vi "get data types of channels.vi"(8 "error in (no error)":errorcluster, 11 "channels in":refnum<class "TBM channel.lvclass">[](array[class])) -> (0 "error out":errorcluster, 2 "data types":T1[](array[typedef]), 3 "channels out":refnum<class "TBM channel.lvclass">[](array[class]))   [LabVIEW 2013, in "Shared Memory configuration.lvclass"]
uses:
  Shared Memory configuration.lvclass
  <vilib>/NI/Tag Bus Module Framework/channel/TBM channel.lvclass
  <vilib>/NI/Tag Bus/tag/Data Type.ctl
  <vilib>/NI/Tag Bus/tag/tag descriptor.lvclass/tag descriptor.ctl
  <vilib>/NI/Tag Bus/tag/tag descriptor.lvclass
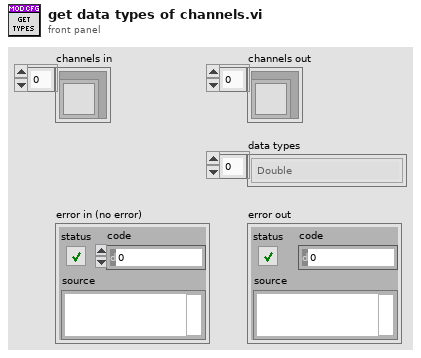
[diagram p1: front panel]
types:
  T1 = typedef "tag bus.lvlib/tag descriptor.lvclass/Data Type.ctl" = enum16{"Double", "Single", "I64", "I32", "I16", "I8", "U64", "U32", "U16", "U8", "Boolean", "String", "Array of Double", "Array of Single", "Array of I64", "Array of I32", "Array of I16", "Array of I8", "Array of U64", "Array of U32", "Array of U16", "Array of U8", "Array of Boolean", "Array of String"}
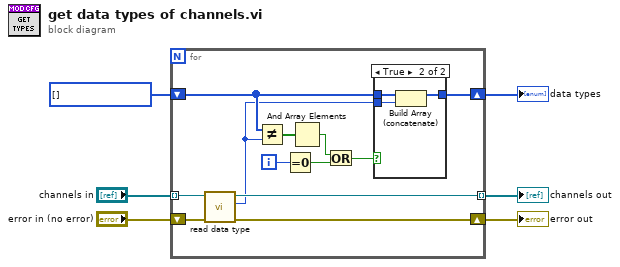
[diagram p0: block diagram]
diagram:
  w2 = T1[] [] items=["Double", "Single", "I64", "I32", "I16", "I8", "U64", "U32", "U16", "U8", "Boolean", "String", "Array of Double", "Array of Single", "Array of I64", "Array of I32", "Array of I16", "Array of I8", "Array of U64", "Array of U32", "Array of U16", "Array of U8", "Array of Boolean", "Array of String"]
  n1 = for {
    tunnel: "channels in" -> [w18] mode=indexing
    shift-right: [w16] -> w4
    shift-left: w2 -> [w15]
    shift-right: [w10] -> w6
    shift-left: "error in (no error)" -> [w9]
    tunnel: [w8] -> w5 mode=indexing
    i -> [w17]
    n2 = call <vilib>:"read data type.vi"("error in"=w9, "system tag in"=w18) -> ("error out"=w10:errorcluster, "data type"=w7:T1, "system tag out"=w8:refnum<class "TBM channel.lvclass">)  [unwired: 7 in]
    n3 = Not Equal?(x=w15, y=w7) -> (x != y?=w14:bool[])
    n4 = Equal To 0?(x=w17) -> (x = 0?=w12:bool)
    n5 = And Array Elements(Boolean array=w14) -> (logical AND=w13:bool)
    n6 = Or(x=w13, y=w12) -> (x .or. y?=w11:bool)
    n7 = case shown="True" w11 {
      tunnel: w15 -> [w19 w22]
      tunnel: [w19 w21] -> w16
      tunnel: w7 -> [_ w20]
      frame False {
      }
      frame True {
        n8 = Build Array (concatenate)(w22, w20) -> (w21:T1[])
      }
    }
  }
  "error out" <- w6
  "channels out" <- w5
  "data types" <- w4
